vi "AddNodeToBranch.vi"(9 "Data":variant, 10 "Unique Node Name":string, 11 "Parent Node In":refnum<data-value>) -> (3 "Parent Node Out":refnum<data-value>)   [LabVIEW 2019]
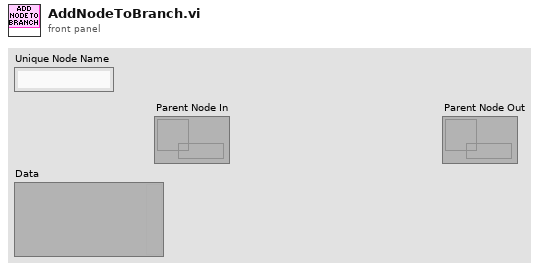
[diagram p1: front panel]
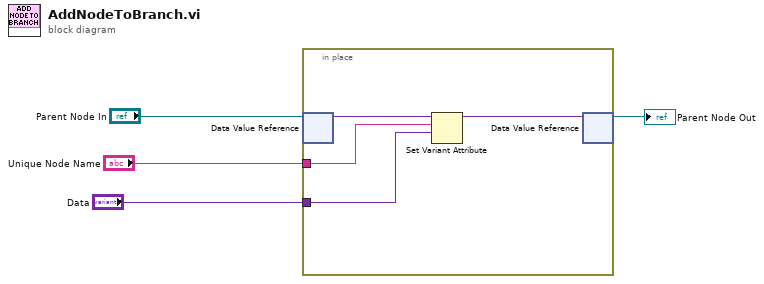
[diagram p0: block diagram]
diagram:
  n1 = in-place {
    in-place-border: "Unique Node Name" -> [w6]
    in-place-border: "Data" -> [w5]
    n2 = in-place-dvr #1("Parent Node In") -> (w8:variant)  [unwired: 1 out]
    n3 = Set Variant Attribute(Variant=w8, name=w6, value=w5) -> (Variant out=w7:variant)  [unwired: 1 in, 2 out]
    n4 = in-place-dvr #1(w7) -> (→"Parent Node Out":refnum<data-value>)  [unwired: 1 out]
  }
